vi "设定sub.vi"(5 "温度阈值":i32, 6 "电源阈值":dbl, 8 "亮度阈值":i32, 10 "环境设定":enum16{"不做控制", "清凉夏日", "温暖冬日", "自定义"}(ring)) -> (1 "输出簇":cluster{"温度阈值":i32, "亮度阈值":i32, "电源阈值":dbl}, 3 "环境设定out":enum16{"不做控制", "清凉夏日", "温暖冬日", "自定义"}(ring))   [LabVIEW 2012]
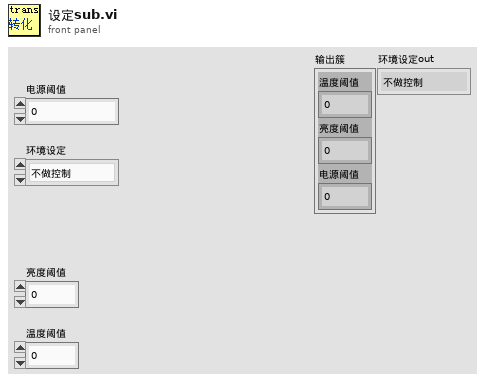
[diagram p1: front panel]
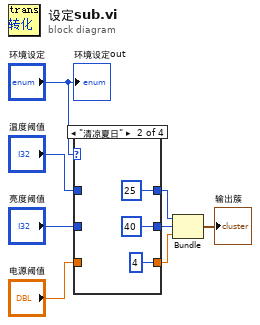
[diagram p0: block diagram]
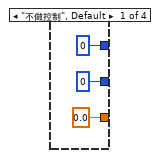
[diagram p2: hidden frame]
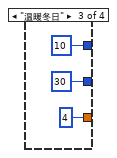
[diagram p3: hidden frame]
diagram:
  n1 = case shown="\"清凉夏日\"" "环境设定" {
    tunnel: [0 ("温度阈值") 25 10 w20] -> w4
    tunnel: [0 ("电源阈值") 40 30 w19] -> w3
    tunnel: "温度阈值" -> [_ _ _ w20]
    tunnel: "亮度阈值" -> [_ _ _ w19]
    tunnel: [0.0 ("电源阈值") 4 4 w18] -> w2
    tunnel: "电源阈值" -> [_ _ _ w18]
    frame "不做控制", Default {
    }
    frame "清凉夏日" {
    }
    frame "温暖冬日" {
    }
    frame "自定义" {
    }
  }
  n2 = Bundle("温度阈值"=w4, "亮度阈值"=w3, "电源阈值"=w2) -> (→"输出簇":cluster{"温度阈值":i32, "亮度阈值":i32, "电源阈值":dbl})  [unwired: 1 in]
  "环境设定out" <- "环境设定"
